vi "File.Delete Files and SubFolders in a Dir.vi"(8 "error in":errorcluster, 9 "Subfolders":bool=TRUE, 10 "Files":bool=TRUE, 11 "Dir":path=path "C:/MTE/Circle Test/Reports/Current Test Data Files") -> (0 "error out":errorcluster, 3 "Dup Dir":path)   [LabVIEW 2024, in "EQMF.lvlib" / "File Utils.lvlib"]
uses:
  File Utils.lvlib
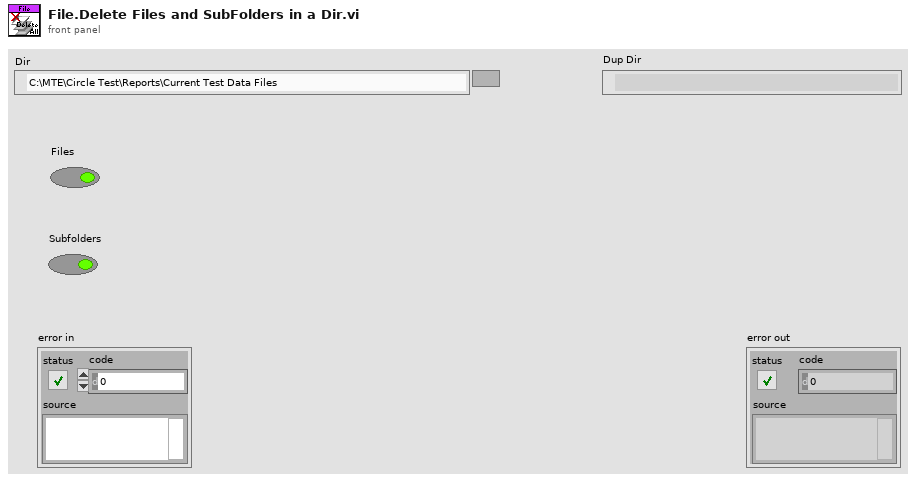
[diagram p1: front panel]
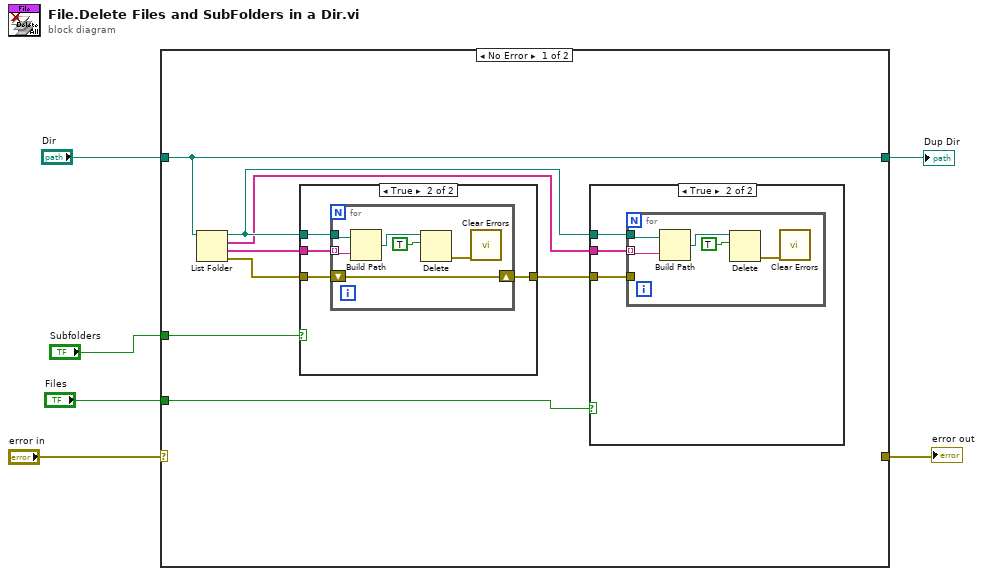
[diagram p0: block diagram]
diagram:
  n1 = case shown="No Error" "error in" {
    selector: "error in" -> [_ w35]
    tunnel: "Dir" -> [w14 w34]
    tunnel: [w14 w34] -> w4
    tunnel: [_ w35] -> w3
    tunnel: "Subfolders" -> [w8 _]
    tunnel: "Files" -> [w7 _]
    frame No Error {
      n2 = List Folder(path=w14) -> (path out=w10:path, filenames=w9:string[], folder names=w13:string[], error out=w12:errorcluster)  [unwired: 3 in]
      n3 = case shown="True" w8 {
        tunnel: w13 -> [_ w27]
        tunnel: w12 -> [w23 w26]
        tunnel: [w23 w25] -> w11
        tunnel: w10 -> [_ w24]
        frame False {
        }
        frame True {
          n4 = for {
            tunnel: w24 -> [w33]
            tunnel: w27 -> [w32] mode=indexing
            shift-right: [w28] -> w25
            shift-left: w26 -> [w28]
            n5 = Build Path(base path=w33, name or relative path=w32) -> (appended path=w31:path)
            n6 = Delete(path (use dialog)=w31, entire hierarchy (F)=TRUE) -> (error out=w29:errorcluster)  [unwired: 3 in, 2 out]
            n7 = call <vilib>:"Clear Errors.vi"("error in (no error)"=w29) -> ()  [unwired: 5 in, 2 out]
          }
        }
      }
      n8 = case shown="True" w7 {
        tunnel: w11 -> [_ w17]
        tunnel: w10 -> [_ w16]
        tunnel: w9 -> [_ w15]
        frame False {
        }
        frame True {
          n9 = for {
            tunnel: w16 -> [w22]
            tunnel: w15 -> [w21] mode=indexing
            tunnel: w17 -> [_]
            n10 = Build Path(base path=w22, name or relative path=w21) -> (appended path=w20:path)
            n11 = Delete(path (use dialog)=w20, entire hierarchy (F)=TRUE) -> (error out=w18:errorcluster)  [unwired: 3 in, 2 out]
            n12 = call <vilib>:"Clear Errors.vi"("error in (no error)"=w18) -> ()  [unwired: 5 in, 2 out]
          }
        }
      }
    }
    frame Error {
    }
  }
  "error out" <- w3
  "Dup Dir" <- w4
